vi "Simple Add.vi"() -> ()   [LabVIEW 2019]
panel:
  in  "Addend3":dbl
  out "Sum":dbl
  in  "Addend2":dbl
  in  "Addend1":dbl
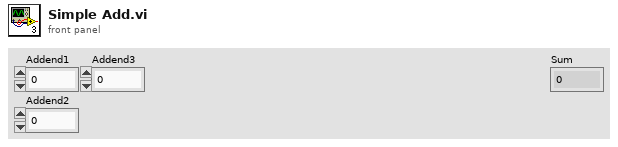
[diagram p1: front panel]
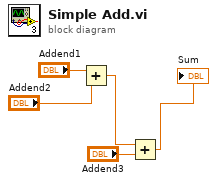
[diagram p0: block diagram]
diagram:
  n1 = Add(x="Addend1", y="Addend2") -> (x+y=w3:dbl)
  n2 = Add(x=w3, y="Addend3") -> (x+y=→"Sum":dbl)
